vi "Begin.vi"() -> (0 "error out":errorcluster, 1 "CameraDevRef":T1)   [LabVIEW 2011]
doc: "Called before other user functions, this VI is expected to open initial I/O refnums, load in file data, and do all program initialization. Notice that the <B>error out</B> terminal is simply used for data flow. Wiring it to other structures or subVIs ensures that this VI runs first."
uses:
  <vilib>/Rock Robotics/WPI/Camera/WPI_CameraDevRef.ctl
  <vilib>/Rock Robotics/SystemInterfaces/DIO/FPGA_DIOPWMChannel.ctl
  <vilib>/Rock Robotics/WPI/Joystick/WPI_JoystickDeviceEnum.ctl
  <vilib>/Rock Robotics/WPI/Relay/WPI_RelayDirection.ctl
  <vilib>/Rock Robotics/SystemInterfaces/DIO/FPGA_DIORelayChannel.ctl
  <vilib>/Rock Robotics/SystemInterfaces/Typedef/FPGA_TypedefDigitalModule.ctl
  <vilib>/Rock Robotics/SystemInterfaces/AI/FPGA_AIChannel.ctl
  <vilib>/Rock Robotics/SystemInterfaces/DIO/FPGA_DIOChannel.ctl
  <vilib>/Rock Robotics/WPI/Encoder/WPI_EncoderType.ctl
  <vilib>/Rock Robotics/WPI/MotorControl/WPI_MotorControlOpen Jaguar.vi
  <vilib>/Rock Robotics/WPI/MotorControl/WPI_MotorControlOpen Victor.vi
  Robot Global Data.vi
  <vilib>/Rock Robotics/WPI/Counter/WPI_CounterDigitalInputToDigitalSource.vi
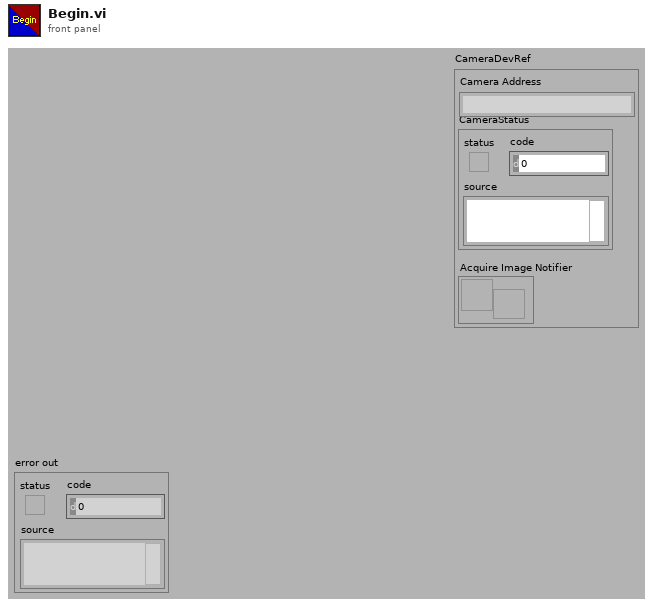
[diagram p1: front panel]
types:
  T1 = typedef "WPI_CameraDevRef.ctl" = cluster{"Camera Address":string, "CameraStatus":errorcluster, "Acquire Image Notifier":refnum<notifier>}
  T2 = typedef "WPI_EncoderType.ctl" = enum16{"1x", "2x", "4x"}
  T3 = typedef "FPGA_DIOChannel.ctl" = enum8{"DIO 1", "DIO 2", "DIO 3", "DIO 4", "DIO 5", "DIO 6", "DIO 7", "DIO 8", "DIO 9", "DIO 10", "DIO 11", "DIO 12", "DIO 13", "DIO 14", "Invalid"}
  T4 = typedef "FPGA_AIChannel.ctl" = enum8{"AI 1", "AI 2", "AI 3", "AI 4", "AI 5", "AI 6", "AI 7", "AI 8", "Invalid"}
  T5 = typedef "FPGA_TypedefDigitalModule.ctl" = enum16{"Digital Module 1", "Digital Module 2"}
  T6 = typedef "FPGA_DIORelayChannel.ctl" = enum8{"Relay 1", "Relay 2", "Relay 3", "Relay 4", "Relay 5", "Relay 6", "Relay 7", "Relay 8", "Invalid"}
  T7 = typedef "WPI_RelayDirection.ctl" = enum16{"Both directions", "Forward only", "Reverse only"}
  T8 = typedef "WPI_JoystickDeviceEnum.ctl" = enum16{"USB 1", "USB 2", "USB 3", "USB 4", "Kinect 1", "Kinect 2"}
  T9 = typedef "FPGA_DIOPWMChannel.ctl" = enum8{"PWM 1", "PWM 2", "PWM 3", "PWM 4", "PWM 5", "PWM 6", "PWM 7", "PWM 8", "PWM 9", "PWM 10", "Invalid"}
  T10 = typedef "WPI_CameraImageSize.ctl" = enum16{"640x480", "320x240", "160x120"}
  T11 = cluster{"fps":i32, "compression":i32, "Image Size":T10}
  T12 = typedef "WPI_DigitalInputDevRef.ctl" = cluster{"DevStatus":errorcluster, "DIO Channel":T3, "Digital Module":T5}
  T13 = typedef "FPGA_CounterEncoderSourceConvertionLVSourceType.ctl" = cluster{"DevStatus":errorcluster, "AnalogTriggerMode?":bool, "DigitalMode":cluster{"Digital Module":T5, "DIO Channel":T14}, "AnalogTriggerMode":cluster{"AnalogTriggerIndex":T15, "OutputType":T16}}
  T14 = typedef "FPGA_DIODigitalSourceChannel.ctl" = enum8{"DIO 1", "DIO 2", "DIO 3", "DIO 4", "DIO 5", "DIO 6", "DIO 7", "DIO 8", "DIO 9", "DIO 10", "DIO 11", "DIO 12", "DIO 13", "DIO 14", "Disabled"}
  T15 = typedef "FPGA_AnalogTriggerIndex.ctl" = enum8{"Trig 0", "Trig 1", "Trig 2", "Trig 3", "Trig 4", "Trig 5", "Trig 6", "Trig 7", "Invalid"}
  T16 = typedef "FPGA_AnalogTriggerOutType.ctl" = enum16{"InWindow", "TriggerState", "Rising", "Falling"}
  T17 = typedef "WPI_EncoderDevRef.ctl" = cluster{"DevStatus":errorcluster, "EncoderIndex":T18, "CounterIndex":T19, "DistancePerCount":dbl, "Decoding Type":T2}
  T18 = typedef "FPGA_EncoderIdx.ctl" = enum8{"Enc 0", "Enc 1", "Enc 2", "Enc 3", "Invalid"}
  T19 = typedef "FPGA_CounterCtrSystemIndex.ctl" = enum8{"Ctr 0", "Ctr 1", "Ctr 2", "Ctr 3", "Ctr 4", "Ctr 5", "Ctr 6", "Ctr 7", "Invalid"}
  T20 = typedef "WPI_CameraWhite Balance Values.ctl" = enum16{"Auto", "Fixed indoor", "Fixed outdoor 1", "Fixed outdoor 2", "Fixed fluorescent 1", "Fixed fluorescent 2", "Hold current"}
  T21 = typedef "WPI_CameraExposure Values.ctl" = enum16{"Auto", "Flicker-free 50 Hz", "Flicker-free 60 Hz", "Hold current"}
  T22 = typedef "WPI_ServoDeviceRef.ctl" = cluster{"DeviceStatus":errorcluster, "Digital Module":T5, "PWM Channel":T9, "DeadBand":T23}
  T23 = typedef "WPI_PWMDeadband.ctl" = cluster{"Name":string, "maxPositivePwm":i32, "minPositivePwm":i32, "centerPwm":i32, "maxNegativePwm":i32, "minNegativePwm":i32, "angularRange":u16}
  T24 = typedef "WPI_MotorControlDeviceRef.ctl" = cluster{"DeviceStatus":errorcluster, "Type":enum16{"PWM", "CAN"}, "PWM":cluster{"Digital Module":T5, "PWM Channel":T9, "DeadBand":T23}, "CAN":cluster{"Device Number":u8, "Control Mode":T25, "Semaphore":T26, "Max Vout":dbl}, "Invert":bool, "TransformRef":T27, "InvTransformRef":T27}
  T25 = typedef "WPI_CANJaguar_ControlMode.ctl" = enum8{"Percent VBus", "Current", "Speed", "Position", "Voltage"}
  T26 = typedef "Semaphore RefNum" = refnum<k1>
  T27 = typedef "WPI_PWMTransform_ConPane.ctl" = refnum<vi>
  T28 = typedef "WPI_AnalogChannelDevRef.ctl" = cluster{"DevStatus":errorcluster, "Analog Module":T29, "Analog Channel":T4}
  T29 = typedef "FPGA_TypedefAnalogModule.ctl" = enum16{"Analog Module 1", "Analog Module 2"}
  T30 = typedef "WPI_JoystickDevRef.ctl" = cluster{"Device":T8}
  T31 = typedef "WPI_RelayDevRef.ctl" = cluster{"DevStatus":errorcluster, "Relay Channel":T6, "Digital Module":T5, "Relay Direction":T7}
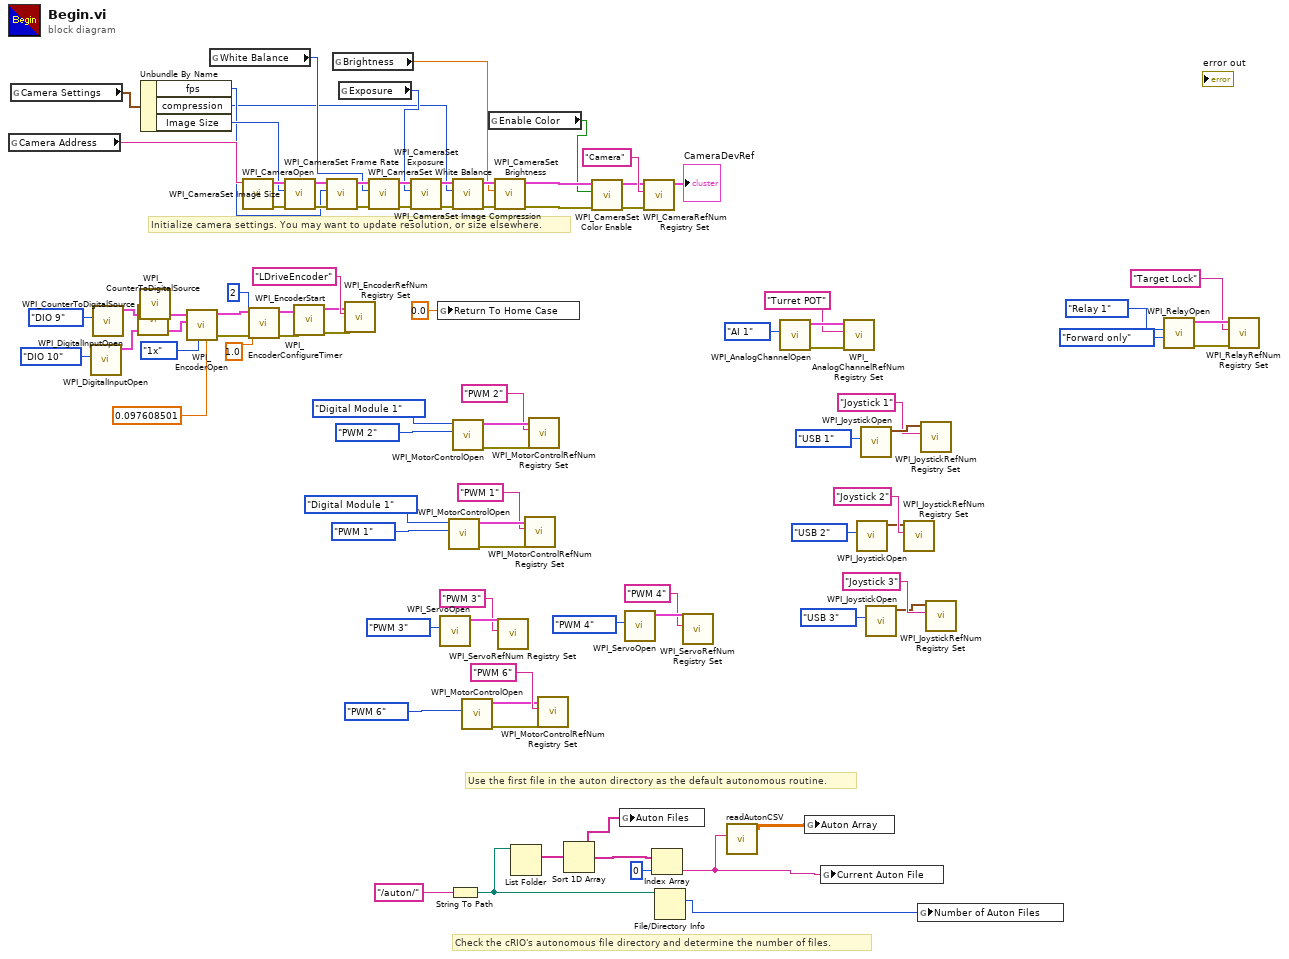
[diagram p0: block diagram]
diagram:
  # "Check the cRIO's autonomous file directory and determine the number of files."
  # "Use the first file in the auton directory as the default autonomous routine."
  # "Initialize camera settings. You may want to update resolution, or size elsewhere."
  n1 = global read "Robot Global Data.vi" "Camera Address"() -> (w78:string)
  n2 = global read "Robot Global Data.vi" "Camera Settings"() -> (w50:T11)
  n3 = call <vilib>:"WPI_DigitalInputOpen.vi"("DIO Channel"=FPGA_DIOChannel."DIO 10") -> ("DigitalInputDevRef"=w13:T12)  [unwired: 9 in, 1 out]
  n4 = call <vilib>:"WPI_DigitalInputOpen.vi"("DIO Channel"=FPGA_DIOChannel."DIO 9") -> ("DigitalInputDevRef"=w16:T12)  [unwired: 9 in, 1 out]
  n5 = call-poly <vilib>:"WPI_CounterToDigitalSource.vi"("DigitalInputDevRef"=w13) -> ("Digital Source"=w12:T13)  [unwired: 6 in]
  n6 = call-poly <vilib>:"WPI_CounterToDigitalSource.vi"("DigitalInputDevRef"=w16) -> ("Digital Source"=w17:T13)  [unwired: 6 in]
  n7 = Unbundle By Name(w50) -> ("fps"=w48:i32, "compression"=w45:i32, "Image Size"=w49:T10)
  n8 = call <vilib>:"WPI_EncoderOpen.vi"("DistancePerCount"=0.097608501, "Decoding Type"=WPI_EncoderType."1x", "BSource"=w12, "ASource"=w17) -> ("error out"=w8:errorcluster, "EncoderDevRef"=w7:T17)  [unwired: 6 in]
  n9 = global read "Robot Global Data.vi" "White Balance"() -> (w47:T20)
  n10 = call <vilib>:"WPI_CameraOpen.vi"("Camera Address"=w78) -> ("error out"=w84:errorcluster, "CameraDevRef"=w85:T1)  [unwired: 1 in, 8 out]
  n11 = call <vilib>:"WPI_EncoderConfigureTimer.vi"("error in (no error)"=w8, "Number Samples to Average"=u8 2, "Minimum Rate"=1.0, "EncoderDevRef"=w7) -> ("error out"=w3:errorcluster, "EncoderDevRef"=w4:T17)  [unwired: 6 in]
  n12 = call <vilib>:"WPI_CameraSet Image Size.vi"("error in (no error)"=w84, "Image Size"=w49, "CameraDevRef"=w85) -> ("error out"=w83:errorcluster, "CameraDevRef Out"=w86:T1)  [unwired: 7 out]
  n13 = call <vilib>:"WPI_EncoderStart.vi"("error in (no error)"=w3, "EncoderDevRef"=w4) -> ("error out"=w1:errorcluster, "EncoderDevRef"=w2:T17)  [unwired: 8 in]
  n14 = call <vilib>:"WPI_CameraSet Frame Rate.vi"("error in (no error)"=w83, "Frame Rate (fps)"=w48, "CameraDevRef"=w86) -> ("error out"=w82:errorcluster, "CameraDevRef Out"=w88:T1)  [unwired: 7 out]
  n15 = global read "Robot Global Data.vi" "Brightness"() -> (w44:dbl)
  n16 = global read "Robot Global Data.vi" "Exposure"() -> (w46:T21)
  n17 = call <vilib>:"WPI_EncoderRefNum Registry Set.vi"("error in (no error)"=w1, "refnum name"="LDriveEncoder", "EncoderDevRef"=w2) -> ()  [unwired: 7 in, 2 out]
  n18 = call <vilib>:"WPI_CameraSet White Balance.vi"("error in (no error)"=w82, "White Balance"=w47, "CameraDevRef"=w88) -> ("error out"=w81:errorcluster, "CameraDevRef Out"=w87:T1)  [unwired: 7 out]
  n19 = call <vilib>:"WPI_CameraSet Exposure.vi"("error in (no error)"=w81, "Exposure"=w46, "CameraDevRef"=w87) -> ("error out"=w80:errorcluster, "CameraDevRef Out"=w90:T1)  [unwired: 7 out]
  n20 = global write "Robot Global Data.vi" "Return To Home Case"(0.0 ("Return To Home Case")) -> ()
  n21 = call <vilib>:"WPI_ServoOpen.vi"("PWM Channel"=FPGA_DIOPWMChannel."PWM 3") -> ("ServoDeviceRef"=w64:T22)  [unwired: 9 in, 1 out]
  n22 = call-poly <vilib>:"WPI_MotorControlOpen.vi"("PWM Channel"=FPGA_DIOPWMChannel."PWM 1", "Digital Module (Module 1)"=FPGA_TypedefDigitalModule."Digital Module 1") -> ("error out"=w70:errorcluster, "MotorControlDeviceRef"=w73:T24)  [unwired: 8 in]
  n23 = String To Path(string="/auton/") -> (path=w24:path)
  n24 = call <vilib>:"WPI_CameraSet Image Compression.vi"("error in (no error)"=w80, "Compression"=w45, "CameraDevRef"=w90) -> ("error out"=w79:errorcluster, "CameraDevRef Out"=w89:T1)  [unwired: 7 out]
  n25 = call-poly <vilib>:"WPI_MotorControlOpen.vi"("PWM Channel"=FPGA_DIOPWMChannel."PWM 2", "Digital Module (Module 1)"=FPGA_TypedefDigitalModule."Digital Module 1") -> ("error out"=w71:errorcluster, "MotorControlDeviceRef"=w76:T24)  [unwired: 8 in]
  n26 = call-poly <vilib>:"WPI_MotorControlOpen.vi"("PWM Channel"=FPGA_DIOPWMChannel."PWM 6") -> ("error out"=w59:errorcluster, "MotorControlDeviceRef"=w57:T24)  [unwired: 9 in]
  n27 = global read "Robot Global Data.vi" "Enable Color"() -> (w39:bool)
  n28 = call <vilib>:"WPI_CameraSet Brightness.vi"("error in (no error)"=w79, "Brightness"=w44, "CameraDevRef"=w89) -> ("error out"=w42:errorcluster, "CameraDevRef Out"=w43:T1)  [unwired: 7 out]
  n29 = call <vilib>:"WPI_ServoRefNum Registry Set.vi"("refnum name"="PWM 3", "ServoDeviceRef"=w64) -> ()  [unwired: 8 in, 2 out]
  n30 = List Folder(path=w24) -> (filenames=w23:string[])  [unwired: 1 in, 5 out]
  n31 = call <vilib>:"WPI_MotorControlRefNum Registry Set.vi"("error in (no error)"=w70, "refnum name"="PWM 1", "MotorControlDevRef"=w73) -> ()  [unwired: 7 in, 2 out]
  n32 = call <vilib>:"WPI_MotorControlRefNum Registry Set.vi"("error in (no error)"=w71, "refnum name"="PWM 2", "MotorControlDevRef"=w76) -> ()  [unwired: 7 in, 2 out]
  n33 = call <vilib>:"WPI_MotorControlRefNum Registry Set.vi"("error in (no error)"=w59, "refnum name"="PWM 6", "MotorControlDevRef"=w57) -> ()  [unwired: 7 in, 2 out]
  n34 = Sort 1D Array(array=w23) -> (sorted array=w18:string[])
  n35 = call <vilib>:"WPI_CameraSet Color Enable.vi"("error in (no error)"=w42, "Color Enabled"=w39, "CameraDevRef"=w43) -> ("error out"=w40:errorcluster, "CameraDevRef Out"=w41:T1)  [unwired: 7 in]
  n36 = global write "Robot Global Data.vi" "Auton Files"(w18) -> ()
  n37 = call <vilib>:"WPI_ServoOpen.vi"("PWM Channel"=FPGA_DIOPWMChannel."PWM 4") -> ("ServoDeviceRef"=w62:T22)  [unwired: 9 in, 1 out]
  n38 = call <vilib>:"WPI_CameraRefNum Registry Set.vi"("error in (no error)"=w40, "refnum name"="Camera", "CameraDevRef"=w41) -> ("CameraDevRef"=→"CameraDevRef":T1)  [unwired: 8 out]
  n39 = Index Array(array=w18, index=0) -> (element=w20:string)
  n40 = File/Directory Info(path=w24) -> (size=w21:i64)  [unwired: 1 in, 6 out]
  n41 = call <vilib>:"WPI_ServoRefNum Registry Set.vi"("refnum name"="PWM 4", "ServoDeviceRef"=w62) -> ()  [unwired: 8 in, 2 out]
  n42 = call "readAutonCSV.vi"("AutonFile"=w20) -> ("AutonArray"=w19:dbl[][])  [unwired: 7 in]
  n43 = call <vilib>:"WPI_AnalogChannelOpen.vi"("Analog Channel"=FPGA_AIChannel."AI 1") -> ("error out"=w29:errorcluster, "AIDeviceRef"=w30:T28)  [unwired: 9 in]
  n44 = global write "Robot Global Data.vi" "Auton Array"(w19) -> ()
  n45 = global write "Robot Global Data.vi" "Current Auton File"(w20) -> ()
  n46 = call <vilib>:"WPI_AnalogChannelRefNum Registry Set.vi"("error in (no error)"=w29, "refnum name"="Turret POT", "AIDeviceRef"=w30) -> ()  [unwired: 7 in, 2 out]
  n47 = call <vilib>:"WPI_JoystickOpen.vi"("JoystickDevice"=WPI_JoystickDeviceEnum."USB 2") -> ("JoystickDevRef"=w66:T30)  [unwired: 10 in]
  n48 = call <vilib>:"WPI_JoystickOpen.vi"("JoystickDevice"=WPI_JoystickDeviceEnum."USB 1") -> ("JoystickDevRef"=w69:T30)  [unwired: 10 in]
  n49 = call <vilib>:"WPI_JoystickOpen.vi"("JoystickDevice"=WPI_JoystickDeviceEnum."USB 3") -> ("JoystickDevRef"=w54:T30)  [unwired: 10 in]
  n50 = call <vilib>:"WPI_JoystickRefNum Registry Set.vi"("refnum name"="Joystick 2", "JoystickDevRef"=w66) -> ()  [unwired: 8 in, 2 out]
  n51 = global write "Robot Global Data.vi" "Number of Auton Files"(w21) -> ()
  n52 = call <vilib>:"WPI_JoystickRefNum Registry Set.vi"("refnum name"="Joystick 1", "JoystickDevRef"=w69) -> ()  [unwired: 8 in, 2 out]
  n53 = call <vilib>:"WPI_JoystickRefNum Registry Set.vi"("refnum name"="Joystick 3", "JoystickDevRef"=w54) -> ()  [unwired: 8 in, 2 out]
  n54 = call <vilib>:"WPI_RelayOpen.vi"("Relay Direction"=WPI_RelayDirection."Forward only", "Relay Channel"=FPGA_DIORelayChannel."Relay 1") -> ("error out"=w36:errorcluster, "RelayDevRef"=w37:T31)  [unwired: 8 in]
  n55 = call <vilib>:"WPI_RelayRefNum Registry Set.vi"("error in (no error)"=w36, "refnum name"="Target Lock", "RelayDevRef"=w37) -> ()  [unwired: 7 in, 2 out]
